vi "BMark_Get Bookmarks.vi"(8 "Error In":errorcluster, 10 "Reset BM Cache?":bool, 11 "App Info":T1) -> (0 "Error Out":errorcluster, 2 "possible undisplayed bookmarks":bool, 3 "bookmarks":T2[](array[typedef]))   [LabVIEW 2018, in "Bookmark Manager.lvlib"]
uses:
  Bookmark Manager.lvlib
  Controls/BMark_Bookmark Data.ctl
  Controls/BMark_VI_Identifier.ctl
  <vilib>/addons/analyzer/_analyzerctrls.llb/VIAnCtl Analysis App Info.ctl
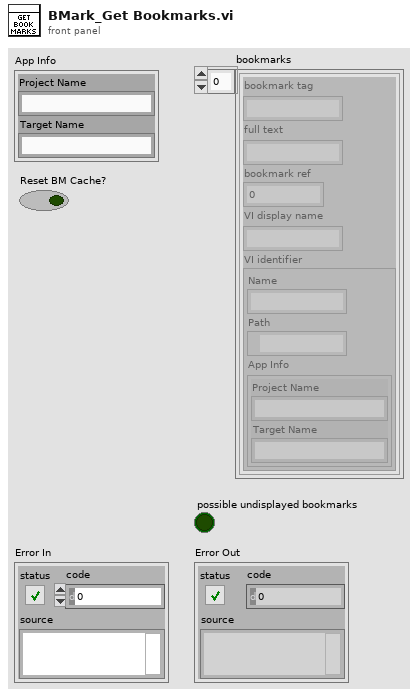
[diagram p1: front panel]
types:
  T1 = typedef "VIAnCtl Analysis App Info.ctl" = cluster{"Project Name":string, "Target Name":string}
  T2 = typedef "Bookmark Manager.lvlib/BMark_Bookmark Data.ctl" = cluster{"bookmark tag":string, "full text":string, "bookmark ref":i32, "VI display name":string, "VI identifier":T3}
  T3 = typedef "Bookmark Manager.lvlib/BMark_VI_Identifier.ctl" = cluster{"Name":string, "Path":path, "App Info":T1}
  T4 = typedef "BMark_VI_Identifier.ctl" = cluster{"Name":string, "Path":path, "App Info":T1}
  T5 = typedef "LVBookmarkInfoTypeDef.ctl" = cluster{"Bookmark ID":u32, "Bookmark Tag":string, "Label Text":string}[]
  T6 = typedef "Bookmark Manager.lvlib/BMark_Array of Bookmarks.ctl" = T7[]
  T7 = typedef "Bookmark Manager.lvlib/BMark_Bookmark Cluster.ctl" = cluster{"bookmark ref":i32, "bookmark":string, "label text":string, "VI identifier":T3}
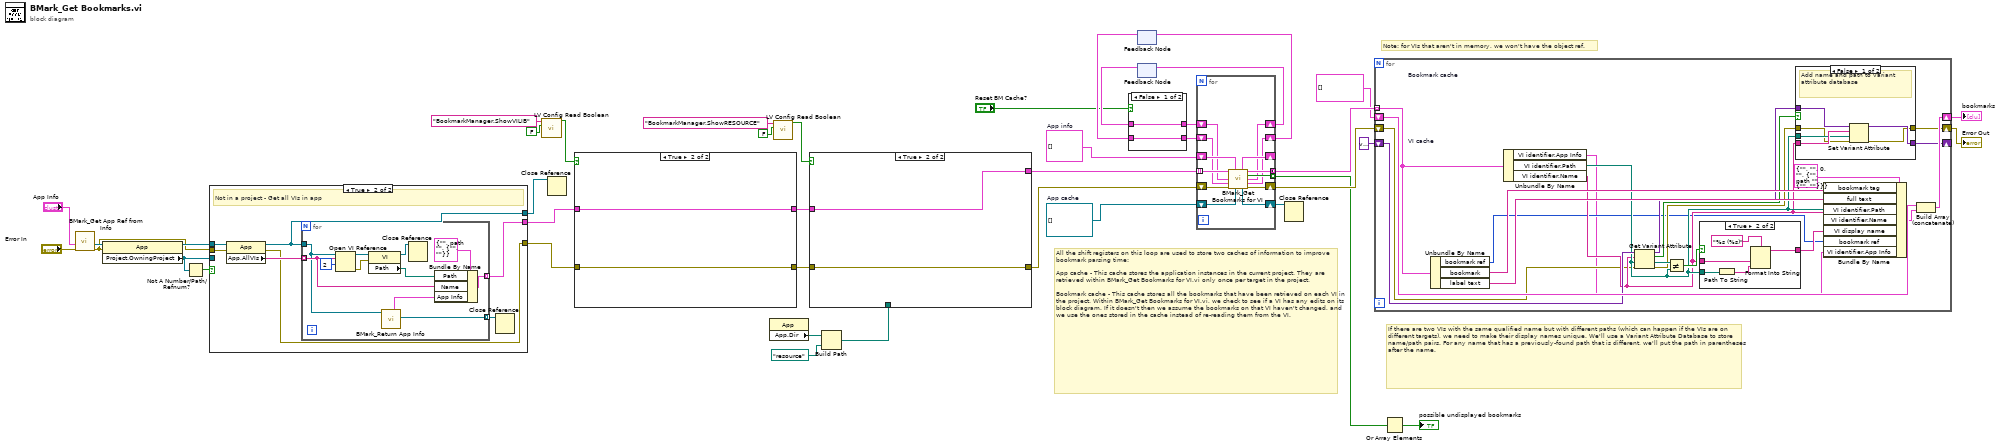
[diagram p0: block diagram]
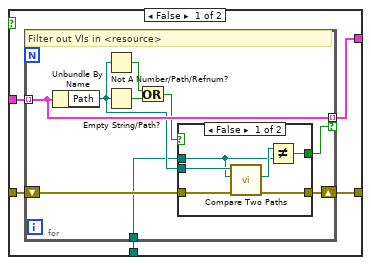
[diagram p3: hidden frame]
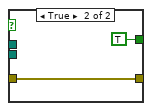
[diagram p4: hidden frame]
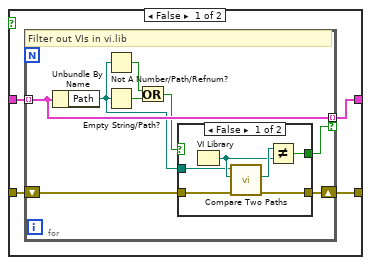
[diagram p5: hidden frame]
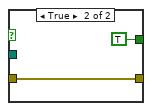
[diagram p6: hidden frame]
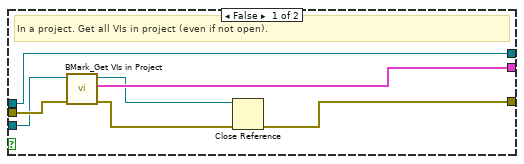
[diagram p7: hidden frame]
diagram:
  w9 = refnum<vi>[] []  # App cache
  w10 = T1[] []  # App info
  # "All the shift registers on this loop are used to store two caches of information to improve bookmark parsing time:\n\nApp cache - This cache stores the application instances in the current project. They are retrieved within BMark_Get Bookmarks for VI.vi only once per target in the project.\n\nBookmark cache - This cache stores all the bookmarks that have been retrieved on each VI in the project. Within BMark_Get Bookmarks for VI.vi, we check to see if a VI has any edits on its block diagram. If it doesn't then we assume the bookmarks on that VI haven't changed, and we use the ones stored in the cache instead of re-reading them from the VI."
  # "Note: for VIs that aren't in memory, we won't have the object ref."
  # "If there are two VIs with the same qualified name but with different paths (which can happen if the VIs are on different targets), we need to make their display names unique. We'll use a Variant Attribute Database to store name/path pairs. For any name that has a previously-found path that is different, we'll put the path in parentheses after the name."
  n1 = call "BMark_Get App Ref from Info.vi"("Error In"="Error In", "Analysis App Info"="App Info") -> ("Error Out"=w25:errorcluster, "Analysis App ref"=w27:refnum<vi>)  [unwired: 8 in]
  n2 = property class="App"(reference=w27, error in=w25) -> (reference out=w39:refnum<vi>, "Project.OwningProject"=w38:refnum<vi>)  [unwired: 1 out]
  n3 = Not A Number/Path/Refnum?(number/path/refnum=w38) -> (NaN/Path/Refnum?=w40:bool)
  n4 = case shown="True" w40 {
    tunnel: w39 -> [w46 w55]
    tunnel: w38 -> [w44 _]
    tunnel: [w42 w51] -> w18
    tunnel: w25 -> [w48 w54]
    tunnel: [w47 w52] -> w17
    tunnel: [w46 w50] -> w24
    frame False {
      # "In a project. Get all VIs in project (even if not open)."
      n5 = call "BMark_Get VIs in Project.vi"("error in (no error)"=w48, "project"=w44) -> ("error out"=w45:errorcluster, "Array of VIs"=w47:T4[], "project out"=w43:refnum<vi>)  [unwired: 7 in]
      n6 = Close Reference(reference=w43, error in (no error)=w45) -> (error out=w42:errorcluster)
    }
    frame True {
      # "Not in a project - Get all VIs in app"
      n7 = property class="App"(reference=w55, error in=w54) -> (reference out=w50:refnum<vi>, error out=w51:errorcluster, "App.AllVIs"=w53:string[])
      n8 = for {
        tunnel: w53 -> [w61] mode=indexing
        tunnel: [w65] -> w52 mode=indexing
        tunnel: w50 -> [w60]
        tunnel: [w57] -> w49 mode=indexing
        n9 = Open VI Reference(application reference (local)=w60, vi path=w61, options=2) -> (vi reference=w64:refnum<vi>, error out=w63:errorcluster)  [unwired: 3 in]
        n10 = property class="VI"(reference=w64, error in=w63) -> (reference out=w58:refnum<vi>, "Path"=w62:path)  [unwired: 1 out]
        n11 = call "BMark_Return App Info.vi"("App Refnum in"=w60) -> ("App Refnum for Opening VI"=w57:refnum<vi>, "App Info"=w59:T1)  [unwired: 8 in, 1 out]
        n12 = Close Reference(reference=w58) -> ()  [unwired: 1 in, 1 out]
        n13 = Bundle By Name(cluster=T3 {"Name"="", "Path"=path "", "App Info"={"Project Name"="", "Target Name"=""}} ("Cluster"), "Path"=w62, "Name"=w61, "App Info"=w59) -> (w65:T3)
      }
      n14 = Close Reference(reference=w49) -> ()  [unwired: 1 in, 1 out]
    }
  }
  n15 = call <resource>:"LV Config Read Boolean.vi"("default value"=FALSE, "key"="BookmarkManager.ShowVILIB") -> ("value"=w32:bool)  [unwired: 3 in, 2 out]
  n16 = Close Reference(reference=w24) -> ()  [unwired: 1 in, 1 out]
  n17 = case shown="True" w32 {
    tunnel: w18 -> [w70 w88]
    tunnel: [w68 w88] -> w22
    tunnel: w17 -> [w69 w87]
    tunnel: [w67 w87] -> w19
    frame False {
      n18 = for {
        shift-right: [w77] -> w68
        shift-left: w70 -> [w78]
        tunnel: w69 -> [w75] mode=indexing
        tunnel: [w75] -> w67 mode=indexing if=w76
        # "Filter out VIs in vi.lib"
        n19 = Unbundle By Name(w75) -> ("Path"=w74:path)
        n20 = Not A Number/Path/Refnum?(number/path/refnum=w74) -> (NaN/Path/Refnum?=w73:bool)
        n21 = Empty String/Path?(string/path=w74) -> (empty?=w72:bool)
        n22 = Or(x=w73, y=w72) -> (x .or. y?=w71:bool)
        n23 = case shown="False" w71 {
          tunnel: w78 -> [w82 w85]
          tunnel: [w81 w85] -> w77
          tunnel: w74 -> [w80 _]
          tunnel: [w79 TRUE] -> w76
          frame False {
            n24 = VI Library() -> (path=w83:path)
            n25 = call <vilib>:"Compare Two Paths.vi"("error in (no error)"=w82, "Path 2"=w83, "Path 1"=w80) -> ("error out"=w81:errorcluster, "Common Path"=w84:path)  [unwired: 5 in, 2 out]
            n26 = Not Equal?(x=w84, y=w83) -> (x != y?=w79:bool)
          }
          frame True {
          }
        }
      }
    }
    frame True {
    }
  }
  n27 = property class="App"() -> ("App.Dir"=w13:path)  [unwired: 2 in, 2 out]
  n28 = call <resource>:"LV Config Read Boolean.vi"("default value"=FALSE, "key"="BookmarkManager.ShowRESOURCE") -> ("value"=w14:bool)  [unwired: 3 in, 2 out]
  n29 = Build Path(base path=w13, name or relative path=path "resource") -> (appended path=w11:path)
  n30 = case shown="True" w14 {
    tunnel: w22 -> [w93 w112]
    tunnel: [w91 w112] -> w21
    tunnel: w19 -> [w92 w111]
    tunnel: [w90 w111] -> w20
    tunnel: w11 -> [w89 _]
    frame False {
      n31 = for {
        shift-right: [w101] -> w91
        shift-left: w93 -> [w102]
        tunnel: w92 -> [w99] mode=indexing
        tunnel: [w99] -> w90 mode=indexing if=w100
        tunnel: w89 -> [w94]
        # "Filter out VIs in <resource>"
        n32 = Unbundle By Name(w99) -> ("Path"=w98:path)
        n33 = Not A Number/Path/Refnum?(number/path/refnum=w98) -> (NaN/Path/Refnum?=w97:bool)
        n34 = Empty String/Path?(string/path=w98) -> (empty?=w96:bool)
        n35 = Or(x=w97, y=w96) -> (x .or. y?=w95:bool)
        n36 = case shown="False" w95 {
          tunnel: w102 -> [w107 w109]
          tunnel: [w106 w109] -> w101
          tunnel: w98 -> [w105 _]
          tunnel: [w104 TRUE] -> w100
          tunnel: w94 -> [w103 _]
          frame False {
            n37 = call <vilib>:"Compare Two Paths.vi"("error in (no error)"=w107, "Path 2"=w103, "Path 1"=w105) -> ("error out"=w106:errorcluster, "Common Path"=w108:path)  [unwired: 5 in, 2 out]
            n38 = Not Equal?(x=w108, y=w103) -> (x != y?=w104:bool)
          }
          frame True {
          }
        }
      }
    }
    frame True {
    }
  }
  n39 = feedback #1 "Bookmark cache"() -> (w3:cluster{"BookmarkInfo":T5}[])  [unwired: 1 in]
  n40 = feedback #2 "VI cache"() -> (w5:T3[])  [unwired: 1 in]
  n41 = case shown="False" "Reset BM Cache?" {
    tunnel: [w114 _] -> w6
    tunnel: w5 -> [w114 _]
    tunnel: [w113 _] -> w4
    tunnel: w3 -> [w113 _]
    frame False {
    }
    frame True {
    }
  }
  n42 = for {
    shift-right: [w126] -> w36
    shift-left: w21 -> [w127]
    tunnel: [w125] -> w37 mode=concatenating
    tunnel: w20 -> [w124] mode=indexing
    tunnel: [w123] -> w30 mode=indexing
    shift-right: [w121] -> _
    shift-left: w10 -> [w122]
    shift-right: [w119] -> w8
    shift-left: w9 -> [w120]
    shift-right: [w118] -> w7
    shift-left: w6 -> [w116]
    shift-right: [w117] -> w1
    shift-left: w4 -> [w115]
    n43 = call "BMark_Get Bookmarks for VI.vi"("VI"=w124, "App Infos in"=w122, "VI Cache in"=w116, "Bookmark Cache in"=w115, "Error In"=w127, "App cache in"=w120) -> ("App Infos out"=w121:T1[], "Array of bookmarks"=w125:T6, "possible undisplayed bookmarks"=w123:bool, "VI Cache out"=w118:T3[], "Bookmark Cache out"=w117:cluster{"BookmarkInfo":T5}[], "App cache out"=w119:refnum<vi>[], "Error Out"=w126:errorcluster)  [unwired: 3 in]
  }
  n44 = feedback-in #1(w1) -> ()
  n45 = feedback-in #2(w7) -> ()
  n46 = Close Reference(reference=w8) -> ()  [unwired: 1 in, 1 out]
  n47 = for {
    shift-right: [w147] -> w41
    shift-left: T2[] [] -> [w148]
    tunnel: w37 -> [w133] mode=indexing
    shift-right: [w134] -> w35
    shift-left: w36 -> [w130]
    shift-right: [w142] -> _
    shift-left: variant -> [w141]
    n48 = Unbundle By Name(w133) -> ("bookmark ref"=w129:i32, "bookmark"=w143:string, "label text"=w144:string)
    n49 = Unbundle By Name(w133) -> ("VI identifier.App Info"=w128:T1, "VI identifier.Path"=w132:path, "VI identifier.Name"=w131:string)
    n50 = Get Variant Attribute(Variant=w141, name=w131, default value (empty Variant)=w132, error in=w130) -> (duplicate Variant=w137:variant, found=w136:bool, value=w140:path, error out=w135:errorcluster)
    n51 = Not Equal?(x=w140, y=w132) -> (x != y?=w138:bool)
    n52 = case shown="True" w138 {
      tunnel: w132 -> [_ w160]
      tunnel: w131 -> [w157 w159]
      tunnel: [w157 w158] -> w139
      frame False {
      }
      frame True {
        n53 = Path To String(path=w160) -> (string=w161:string)
        n54 = Format Into String(format string="%s (%s)", w159, w161) -> (resulting string=w158:string)  [unwired: 2 in, 1 out]
      }
    }
    n55 = case shown="False" w136 {
      tunnel: [w154 w156] -> w142
      tunnel: w137 -> [w153 w156]
      tunnel: w131 -> [w152 _]
      tunnel: w132 -> [w151 _]
      tunnel: w135 -> [w150 w155]
      tunnel: [w149 w155] -> w134
      frame False {
        # "Add name and path to variant attribute database"
        n56 = Set Variant Attribute(Variant=w153, name=w152, value=w151, error in=w150) -> (Variant out=w154:variant, error out=w149:errorcluster)  [unwired: 1 out]
      }
      frame True {
      }
    }
    n57 = Bundle By Name(cluster=T2 {"bookmark tag"="", "full text"="", "bookmark ref"=0, "VI display name"="", "VI identifier"={"Name"="", "Path"=path "", "App Info"={"Project Name"="", "Target Name"=""}}} ("bookmark item"), "bookmark tag"=w143, "full text"=w144, "VI identifier.Path"=w132, "VI identifier.Name"=w131, "VI display name"=w139, "bookmark ref"=w129, "VI identifier.App Info"=w128) -> (w145:T2)
    n58 = Build Array (concatenate)(w148, w145) -> (w147:T2[])
  }
  "bookmarks" <- w41
  "Error Out" <- w35
  n59 = Or Array Elements(Boolean array=w30) -> (logical OR=→"possible undisplayed bookmarks":bool)
